vi "py_add.vi"() -> ()   [LabVIEW 2024]
panel:
  in  "num1 2":dbl format="%#_13g"
  in  "num2 2":dbl format="%#_13g"
  out "ret 2":dbl
  out "ret":dbl
  in  "num2":dbl format="%#_13g"
  in  "num1":dbl format="%#_13g"
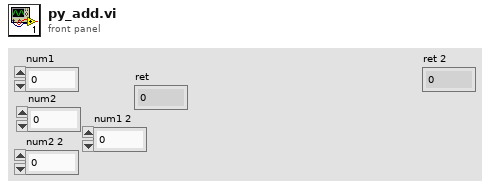
[diagram p1: front panel]
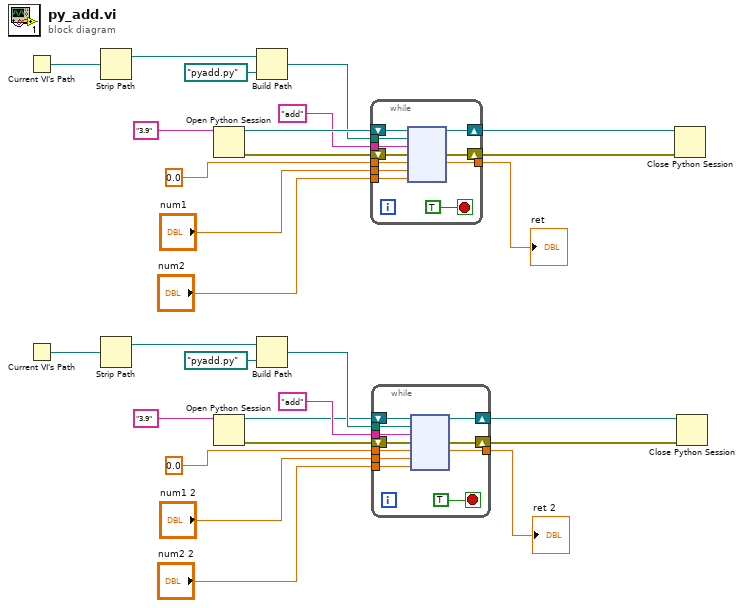
[diagram p0: block diagram]
diagram:
  n1 = Current VI's Path() -> (path=w25:path)
  n2 = Current VI's Path() -> (path=w4:path)
  n3 = Strip Path(path=w25) -> (stripped path=w24:path)  [unwired: 1 out]
  n4 = Strip Path(path=w4) -> (stripped path=w5:path)  [unwired: 1 out]
  n5 = Open Python Session(python version="3.9" ("Python version")) -> (session out=w27:refnum<k35>, error out=w26:errorcluster)  [unwired: 2 in]
  n6 = Open Python Session(python version="3.9" ("Python version")) -> (session out=w2:refnum<k35>, error out=w3:errorcluster)  [unwired: 2 in]
  n7 = Build Path(base path=w24, name or relative path=path "pyadd.py") -> (appended path=w22:path)
  n8 = Build Path(base path=w5, name or relative path=path "pyadd.py") -> (appended path=w7:path)
  n9 = while {
    tunnel: w22 -> [w37]
    tunnel: "add" ("function name") -> [w36]
    tunnel: 0.0 -> [w35]
    tunnel: "num1" -> [w34]
    tunnel: "num2" -> [w33]
    tunnel: [w32] -> w17
    shift-right: [w31] -> w16
    shift-left: w27 -> [w39]
    shift-right: [w30] -> w15
    shift-left: w26 -> [w38]
    stop <- TRUE stop-if-true
    n10 = node(w39, w37, w36, w38, w35, w34, w33) -> (w31:refnum<k35>, w30:errorcluster, w32:dbl)  [unwired: 2 in, 2 out]
  }
  "ret" <- w17
  n11 = while {
    tunnel: [w48] -> w12
    tunnel: "num2 2" -> [w47]
    tunnel: "num1 2" -> [w46]
    tunnel: 0.0 -> [w45]
    tunnel: "add" ("function name") -> [w44]
    tunnel: w7 -> [w43]
    shift-right: [w50] -> w14
    shift-left: w3 -> [w42]
    shift-right: [w49] -> w13
    shift-left: w2 -> [w41]
    stop <- TRUE stop-if-true
    n12 = node(w41, w43, w44, w42, w45, w46, w47) -> (w49:refnum<k35>, w50:errorcluster, w48:dbl)  [unwired: 2 in, 2 out]
  }
  "ret 2" <- w12
  n13 = Close Python Session(session in=w16, error in=w15) -> ()  [unwired: 1 out]
  n14 = Close Python Session(session in=w13, error in=w14) -> ()  [unwired: 1 out]
